vi "Run Step.vi"(8 "error in (no error)":errorcluster, 11 "Plant in":refnum<class "Plant.lvclass">) -> (0 "error out":errorcluster, 3 "Plant out":refnum<class "Plant.lvclass">)   [LabVIEW 2023, in "Plant.lvlib" / "Plant.lvclass"]
uses:
  Plant.lvclass
  Plant.lvclass/Plant.ctl
  <vilib>/addons/control/pid/pid.llb/PID (DBL).vi
  <vilib>/addons/control/pid/NI_PID_pid.lvlib
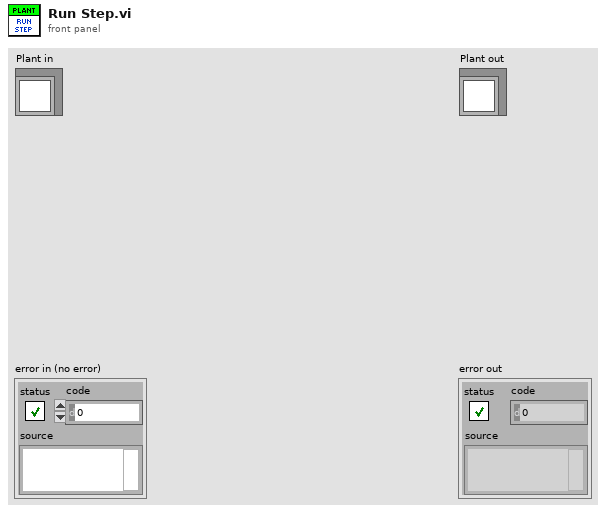
[diagram p1: front panel]
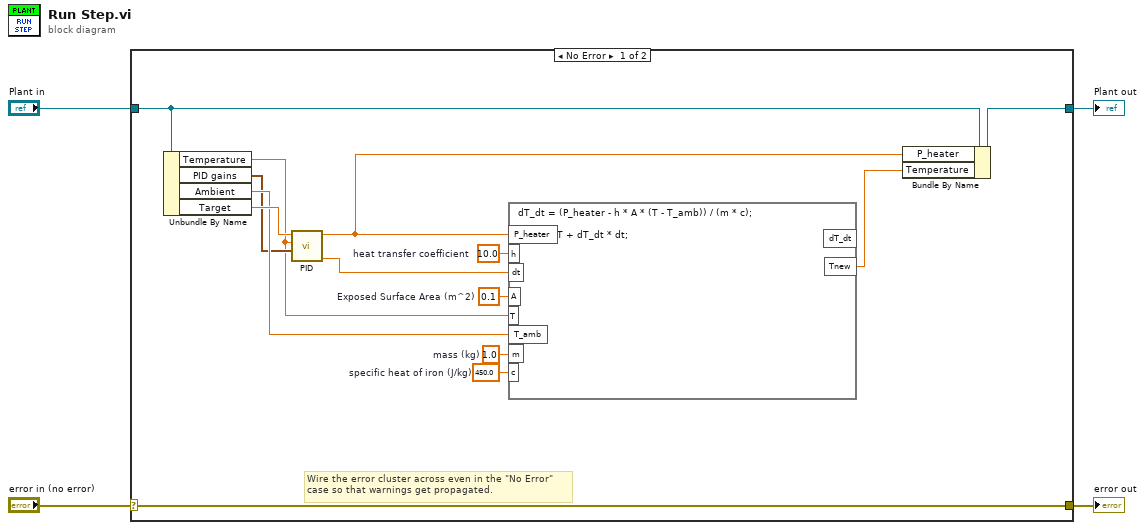
[diagram p0: block diagram]
diagram:
  n1 = case shown="No Error" "error in (no error)" {
    selector: "error in (no error)" -> [w18 w20]
    tunnel: [w18 w20] -> w3
    tunnel: [w5 w19] -> w1
    tunnel: "Plant in" -> [w6 w19]
    frame No Error {
      w13 = 450.0  # specific heat of iron (J/kg)
      w14 = 1.0  # mass (kg)
      w15 = 0.1  # Exposed Surface Area (m^2)
      w16 = 10.0  # heat transfer coefficient
      # "Wire the error cluster across even in the \"No Error\"\ncase so that warnings get propagated."
      n2 = Unbundle By Name(w6) -> ("Temperature"=w7:dbl, "PID gains"=w9:cluster{"P":dbl, "I":dbl, "D":dbl}, "Ambient"=w10:dbl, "Target"=w11:dbl)
      n3 = call-poly <vilib>:"PID.vi"("PID gains"=w9, "process variable"=w7, "setpoint"=w11) -> ("dt out (s)"=w17:dbl, "output"=w12:dbl)  [unwired: 7 in]
      n4 = formula code="dT_dt = (P_heater - h * A * (T - T_amb)) / (m * c);\n\nTnew = T + dT_dt * dt;"("P_heater"=w12, "h"=w16, "A"=w15, "T"=w7, "T_amb"=w10, "m"=w14, "c"=w13, "dt"=w17) -> ("Tnew"=w8:dbl)  [unwired: 1 out]
      n5 = Bundle By Name(cluster=w6, "P_heater"=w12, "Temperature"=w8) -> (w5:refnum<class "Plant.lvclass">)
    }
    frame Error {
    }
  }
  "error out" <- w3
  "Plant out" <- w1
